vi "DataGraph_Set_GraphEnable.vi"(4 "error in (no error)":errorcluster, 5 "Value":bool, 6 "Container State":T2, 7 "Display State In":T1) -> (0 "error out":errorcluster, 3 "Display State Out":T1)   [LabVIEW 2018, in "DataGraphXControl.xctl"]
uses:
  DataGraphXControl.xctl
  <vilib>/_xctls/Container State.ctl
  DataGraph_State.ctl
  <vilib>/_xctls/XControlSupport.lvlib
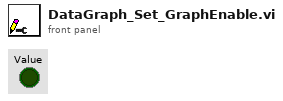
[diagram p1: front panel]
types:
  T1 = typedef "DataGraphXControl.xctl/DataGraph_State.ctl" = cluster{"Mouse State":enum16{"Zoom In", "Select Range"}, "Rectangle X":cluster{"Minimum":dbl, "Maximum":dbl}, "Rectangle Y":cluster{"Minimum":dbl, "Maximum":dbl}, "X Index":cluster{"Minimum":u32, "Maximum":u32}, "FilePath":path, "Allow Index Bool":bool[], "Retangle Enable":bool, "Graph Enable":bool, "Aux Label Enable":bool}
  T2 = typedef "XControlSupport.lvlib/Container State.ctl" = cluster{"Indicator?":bool, "Run Mode?":bool, " Refnum":refnum<vi>}
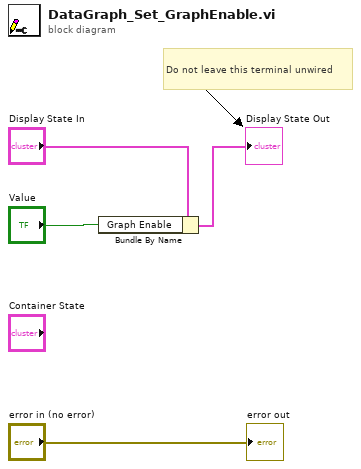
[diagram p0: block diagram]
diagram:
  # "Do not leave this terminal unwired"
  n1 = Bundle By Name(cluster="Display State In", "Graph Enable"="Value") -> (→"Display State Out":T1)
  "error out" <- "error in (no error)"
